vi "断电保存全局变量.vi"() -> ()   [LabVIEW 2016, in "环境动力监测库.lvlib"]
uses:
  <vilib>/Plasmionique/MB Master/MB_Master/MB_Master.lvclass
panel:
  in  "高温告警开关":bool
  in  "湿度下限告警点":dbl
  in  "湿度上限告警点":dbl
  in  "室温下限告警点":dbl
  in  "室温上限告警点":dbl
  out "配置ItemNames":string[][](array[string])
  in  "型号选择":enum16{"黑盾", "英维克"}(ring)
  out "MB session in":refnum<class "MB_Master.lvclass">
  out "英维克空调寄存器":u16[](array[numeric])
  out "通讯状态":bool
  in  "PORT":string="502"
  in  "IP":string="192.168.1.207"
  in  "Slave ID":u8=1
  in  "Serial Config":T1={"baud rate (bps)"=9600, "stop bits"=10, "parity"=0, "flow control"=0, "timeout"=1000, "retries"=1} {"stop bits" items=["1.0"=10, "1.5"=15, "2.0"=20]; "flow control" items=["None", "XON/XOFF", "RTS/CTS", "XON/XOFF & RTS/CTS", "DTR/DSR", "XON/XOFF & DTR/DSR"]; "parity" items=["None", "Odd", "Even", "Mark", "Space"]}
  in  "Error in":errorcluster
  in  "VISA Resource":refnum<visa-resource-name>="COM9"
  in  "MB通信方式选择":enum16{"串口", "TCP"}(ring)
  # "黑盾/英维克空调"
  # "MB串口参数"
  # "MBTCP参数"
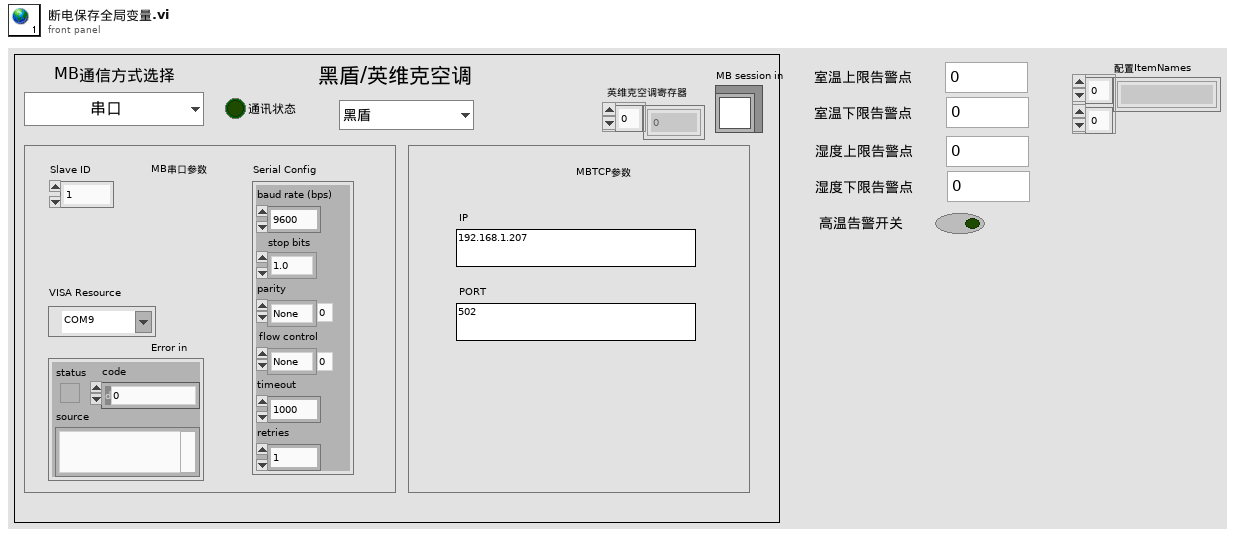
[diagram p1: front panel]
types:
  T1 = cluster{"baud rate (bps)":u32, "stop bits":u16, "parity":u16, "flow control":u16, "timeout":u32, "retries":i32}
diagram:
